vi "newsubvi Robot GoTo Image.vi"(2 "Magnification":u8, 3 "Objective":u8, 4 "VISA In":refnum<visa-resource-name>) -> (0 "error out":errorcluster, 1 "VISA Out":refnum<visa-resource-name>)   [LabVIEW 2012]
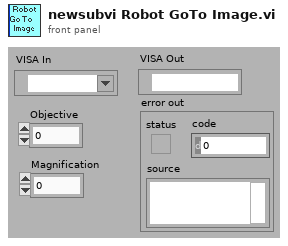
[diagram p1: front panel]
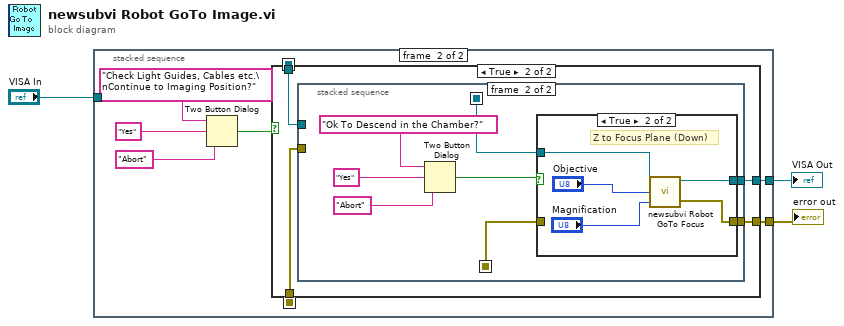
[diagram p0: block diagram]
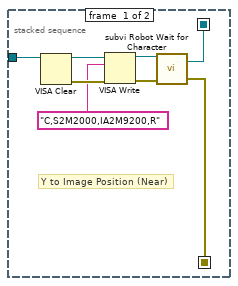
[diagram p2: hidden frame]
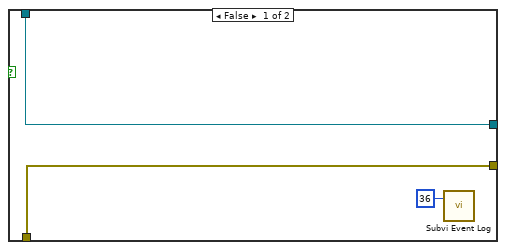
[diagram p3: hidden frame]
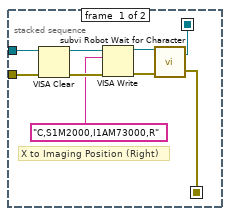
[diagram p4: hidden frame]
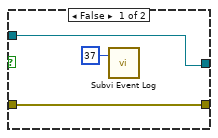
[diagram p5: hidden frame]
diagram:
  n1 = stacked-sequence {
    seq-local: [w5 _] -> [_ w15]
    seq-local: [w4 _] -> [_ w14]
    tunnel: "VISA In" -> [w7 _]
    tunnel: [_ w13] -> w2
    tunnel: [_ w12] -> w1
    frame #0 {
      # "Y to Image Position (Near)"
      n2 = VISA Clear(VISA resource name=w7) -> (VISA resource name out=w11:refnum<visa-resource-name>, error out=w10:errorcluster)  [unwired: 1 in]
      n3 = VISA Write(VISA resource name=w11, write buffer="C,S2M2000,IA2M9200,R" ("Text to Send"), error in (no error)=w10) -> (VISA resource name out=w9:refnum<visa-resource-name>, error out=w8:errorcluster)  [unwired: 1 out]
      n4 = call "subvi Robot Wait for Character.vi"("error in"=w8, "VISA In"=w9) -> ("error out"=w4:errorcluster, "VISA Out"=w5:refnum<visa-resource-name>)
    }
    frame #1 {
      n5 = Two Button Dialog(message="Check Light Guides, Cables etc.\nContinue to Imaging Position?", 1:"Abort" ("F button name (\"Cancel\")"), 2:"Yes" ("T button name (\"OK\")")) -> (T button?=w16:bool)
      n6 = case shown="True" w16 {
        tunnel: w15 -> [w21 w26]
        tunnel: w14 -> [w20 w25]
        tunnel: [w21 w24] -> w13
        tunnel: [w20 w23] -> w12
        frame False {
          n7 = call "Subvi Event Log.vi"("EventNum"=u32 36) -> ()  [unwired: 1 in]
        }
        frame True {
          n8 = stacked-sequence {
            seq-local: [w28 _] -> [_ w39]
            seq-local: [w27 _] -> [_ w36]
            tunnel: w26 -> [w31 _]
            tunnel: w25 -> [w30 _]
            tunnel: [_ w38] -> w24
            tunnel: [_ w37] -> w23
            frame #0 {
              # "X to Imaging Position (Right)"
              n9 = VISA Clear(VISA resource name=w31, error in (no error)=w30) -> (VISA resource name out=w35:refnum<visa-resource-name>, error out=w34:errorcluster)
              n10 = VISA Write(VISA resource name=w35, write buffer="C,S1M2000,I1AM73000,R" ("Text to Send"), error in (no error)=w34) -> (VISA resource name out=w33:refnum<visa-resource-name>, error out=w32:errorcluster)  [unwired: 1 out]
              n11 = call "subvi Robot Wait for Character.vi"("error in"=w32, "VISA In"=w33) -> ("error out"=w27:errorcluster, "VISA Out"=w28:refnum<visa-resource-name>)
            }
            frame #1 {
              n12 = Two Button Dialog(message="Ok To Descend in the Chamber?", 1:"Abort" ("F button name (\"Cancel\")"), 2:"Yes" ("T button name (\"OK\")")) -> (T button?=w40:bool)
              n13 = case shown="True" w40 {
                tunnel: w39 -> [w45 w49]
                tunnel: [w45 w48] -> w38
                tunnel: [w44 w47] -> w37
                tunnel: w36 -> [w44 _]
                frame False {
                  n14 = call "Subvi Event Log.vi"("EventNum"=u32 37) -> ()  [unwired: 1 in]
                }
                frame True {
                  # "Z to Focus Plane (Down)"
                  n15 = call "newsubvi Robot GoTo Focus.vi"("Magnification"="Magnification", "Objective"="Objective", "VISA In"=w49) -> ("error out"=w47:errorcluster, "VISA Out"=w48:refnum<visa-resource-name>)
                }
              }
            }
          }
        }
      }
    }
  }
  "VISA Out" <- w2
  "error out" <- w1
